vi "TcpCommunicationServerLoop.vi"(8 "エラー入力（エラーなし）":errorcluster, 11 "ポート":u16) -> (0 "エラー出力":errorcluster)   [LabVIEW 2021]
doc: "TCP通信のサーバー機能を提供します。\n停止：TcpCommunicationServerModule.viのStopコマンドを実行することで停止します。\n送信：メッセージの送信はSendListFGV.viに送り先のアドレスと文字列Dataを追加します。\n受信：受信したメッセージはReadListFGV.viに格納します。"
uses:
  TcpCommunicationServerCMD.ctl
panel:
  out "接続数":i32
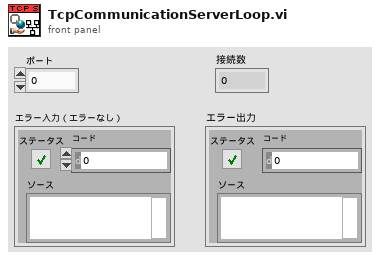
[diagram p1: front panel]
types:
  T1 = typedef "TcpCommunicationServerCMD.ctl" = enum16{"Initialize", "Status Check", "Send Data", "Read Data", "Stop", "GetData"}
  T2 = typedef "TcpCommunicationServerData.ctl" = cluster{"クライアント":refnum<k5>[], "リスナ":refnum<k5>, "リモートアドレス":string[], "SendData":string[]}
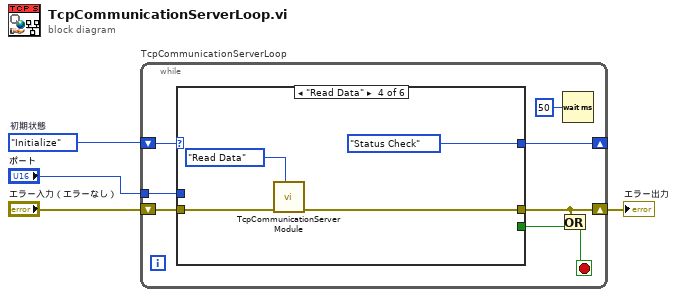
[diagram p0: block diagram]
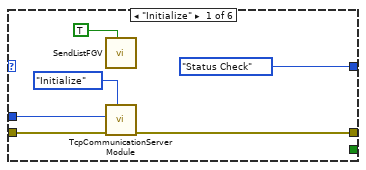
[diagram p2: hidden frame]
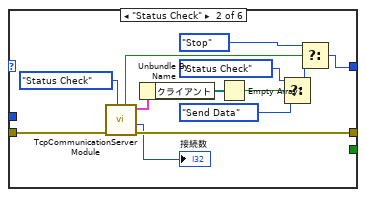
[diagram p3: hidden frame]
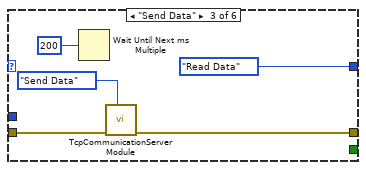
[diagram p4: hidden frame]
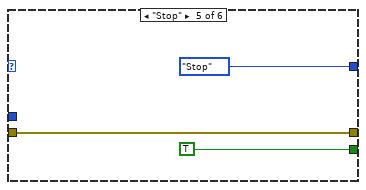
[diagram p5: hidden frame]
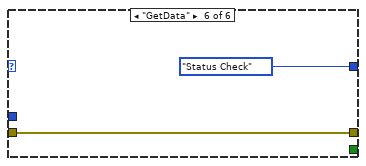
[diagram p6: hidden frame]
diagram:
  w1 = TcpCommunicationServerCMD."Initialize"  # 初期状態
  n1 = while "TcpCommunicationServerLoop" {
    shift-right: [w11] -> _
    shift-left: w1 -> [w12]
    shift-right: [w7] -> w3
    shift-left: "エラー入力（エラーなし）" -> [w10]
    tunnel: "ポート" -> [w6]
    stop <- w8 stop-if-true
    # "TCP複数の接続 - サーバステートマシン"
    n2 = case shown="\"Read Data\"" w12 {
      tunnel: [TcpCommunicationServerCMD."Status Check" ("States") w26 TcpCommunicationServerCMD."Read Data" ("States") TcpCommunicationServerCMD."Status Check" ("States") TcpCommunicationServerCMD."Stop" ("（値未使用）") TcpCommunicationServerCMD."Status Check" ("（値未使用）")] -> w11
      tunnel: [_ _ _ _ TRUE ("ループを停止?") _] -> w9
      tunnel: w10 -> [w18 w24 w34 w38 w41 w45]
      tunnel: [w17 w21 w33 w37 w41 w45] -> w7
      tunnel: w6 -> [w13 _ _ _ _ _]
      frame "Initialize" {
        # "「TCPリスナを作成」関数は、新しいクライアント接続の確認に使用するリスナリファレンスを作成します。"
        n3 = call "SendListFGV.vi"("Set"=TRUE) -> ()  [unwired: 8 in, 3 out]
        n4 = call "TcpCommunicationServerModule.vi"("States"=TcpCommunicationServerCMD."Initialize", "エラー入力（エラーなし）"=w18, "ポート"=w13) -> ("エラー出力"=w17:errorcluster)  [unwired: 5 in, 3 out]
      }
      frame "Status Check" {
        # "停止ボタンのステータスとデータが必要な接続されたクライアントが存在するかどうかを確認します。"
        n5 = call "TcpCommunicationServerModule.vi"("States"=TcpCommunicationServerCMD."Status Check", "エラー入力（エラーなし）"=w24) -> ("エラー出力"=w21:errorcluster, "接続数"=→"接続数":i32, "Data出力"=w23:T2, "Stoped"=w20:bool)  [unwired: 6 in]
        n6 = Unbundle By Name(w23) -> ("クライアント"=w28:refnum<k5>[])
        n7 = Empty Array?(array=w28) -> (empty?=w29:bool)
        n8 = Select(t=TcpCommunicationServerCMD."Status Check" ("States"), s=w29, f=TcpCommunicationServerCMD."Send Data" ("States")) -> (s? t:f=w27:T1)
        n9 = Select(t=TcpCommunicationServerCMD."Stop", s=w20, f=w27) -> (s? t:f=w26:T1)
      }
      frame "Send Data" {
        # "クライアント配列の各項目で以下を実行:\n(1) 「TCP読み取り」関数でクライアントからのバイトを読み取ります。タイムアウトまたは接続が閉じられている場合はエラーを無視します。クライアントからバイトが返された場合は、接続が閉じられていることを意味します。\n(2) エラーがなく、クライアントからバイトが返されなかった場合は、TCP書き込み関数を使って現在のデータ値をクライアントに送信します。"
        n10 = Wait Until Next ms Multiple(millisecond multiple=u32 200 ("ミリ秒倍数")) -> ()  [unwired: 1 out]
        n11 = call "TcpCommunicationServerModule.vi"("States"=TcpCommunicationServerCMD."Send Data", "エラー入力（エラーなし）"=w34) -> ("エラー出力"=w33:errorcluster)  [unwired: 6 in, 3 out]
      }
      frame "Read Data" {
        # "クライアント配列の各項目で以下を実行:\n(1) 「TCP読み取り」関数でクライアントからのバイトを読み取ります。タイムアウトまたは接続が閉じられている場合はエラーを無視します。クライアントからバイトが返された場合は、接続が閉じられていることを意味します。\n(2) エラーがなく、クライアントからバイトが返されなかった場合は、TCP書き込み関数を使って現在のデータ値をクライアントに送信します。"
        n12 = call "TcpCommunicationServerModule.vi"("States"=TcpCommunicationServerCMD."Read Data", "エラー入力（エラーなし）"=w38) -> ("エラー出力"=w37:errorcluster)  [unwired: 6 in, 3 out]
      }
      frame "Stop" {
        # "「TCP接続を閉じる」関数を使用して、すべてのクライアント接続とリスナ接続を閉じます。"
      }
      frame "GetData" {
      }
    }
    n13 = Or(x=w7, y=w9) -> (x .or. y?=w8:bool)
    n14 = Wait (ms)(milliseconds to wait=u32 50 ("ミリ秒待機時間")) -> ()  [unwired: 1 out]
  }
  "エラー出力" <- w3
